vi "runtest initialize fields.vi"(4 "Process SPARTAN SN (F)":bool, 6 "User/Station":T8, 7 "POST (empty)":T6, 8 "error in (no error)":errorcluster, 9 "ProcessNextItem? (f)":bool, 10 "Test Sequence ID":string, 11 "Connection Refnum":T7) -> (0 "error out":errorcluster, 1 "Fields / Results":T5, 2 "dup Test Sequence ID":string, 3 "Connection Refnum":T7, 5 "POST out":T6)   [LabVIEW 2011]
uses:
  Addons/internet/utils/keyedarr.llb/Keyed Array.ctl
  SI.LIB/ODBC/SQL Controls/Connection Refnum.ctl
  runtest User - Station.ctl
  server/database/Stations/Instruments/Instrument Record.ctl
  server/database/Stations/Step Associations/Step Association Record.ctl
  server/database/Fields/Field Record.ctl
  server/database/Fields/Field DataTypes.ctl
  server/database/Fields/Field NextItem.ctl
  tests/Test Output.ctl
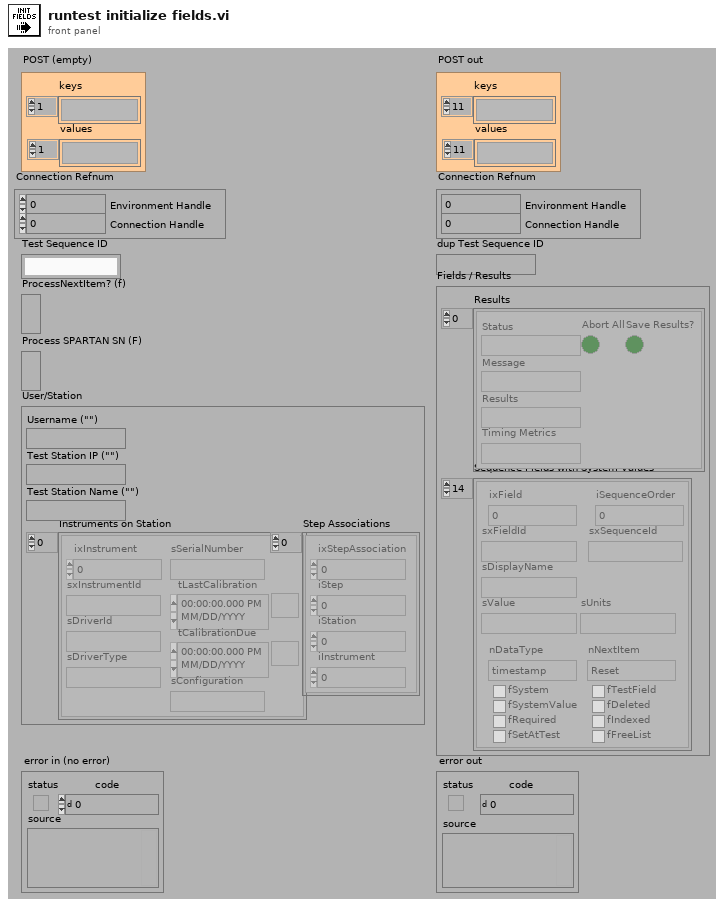
[diagram p1: front panel]
types:
  T1 = typedef "Field Record.ctl" = cluster{"ixField":i32, "iSequenceOrder":i32, "sxFieldId":string, "sxSequenceId":string, "sDisplayName":string, "sValue":string, "sUnits":string, "nDataType":T2, "nNextItem":T3, "fSystem":bool, "fSystemValue":bool, "fRequired":bool, "fSetAtTest":bool, "fTestField":bool, "fDeleted":bool, "fIndexed":bool, "fFreeList":bool}
  T2 = typedef "Field DataTypes.ctl" = enum32{"text", "numeric", "list", "timestamp", "boolean"}
  T3 = typedef "Field NextItem.ctl" = enum32{"Reset", "Retain", "Auto-Increment"}
  T4 = typedef "Test Output.ctl" = cluster{"Status":string, "Message":string, "Results":string, "Abort All":bool, "Save Results?":bool, "Timing Metrics":string}
  T5 = cluster{"Sequence Fields with System Values":T1[], "Results":T4[]}
  T6 = typedef "Keyed Array.ctl" = cluster{"keys":string[], "values":string[]}
  T7 = typedef "Connection Refnum.ctl" = cluster{"Environment Handle":i32, "Connection Handle":i32}
  T8 = typedef "runtest User - Station.ctl" = cluster{"Username (\"\")":string, "Test Station IP (\"\")":string, "Test Station Name (\"\")":string, "Instruments on Station":T9[], "Step Associations":T10[]}
  T9 = typedef "Instrument Record.ctl" = cluster{"ixInstrument":i32, "sxInstrumentId":string, "sDriverId":string, "sDriverType":string, "sSerialNumber":string, "tLastCalibration":timestamp, "tCalibrationDue":timestamp, "sConfiguration":string}
  T10 = typedef "Step Association Record.ctl" = cluster{"ixStepAssociation":i32, "iStep":i32, "iStation":i32, "iInstrument":i32}
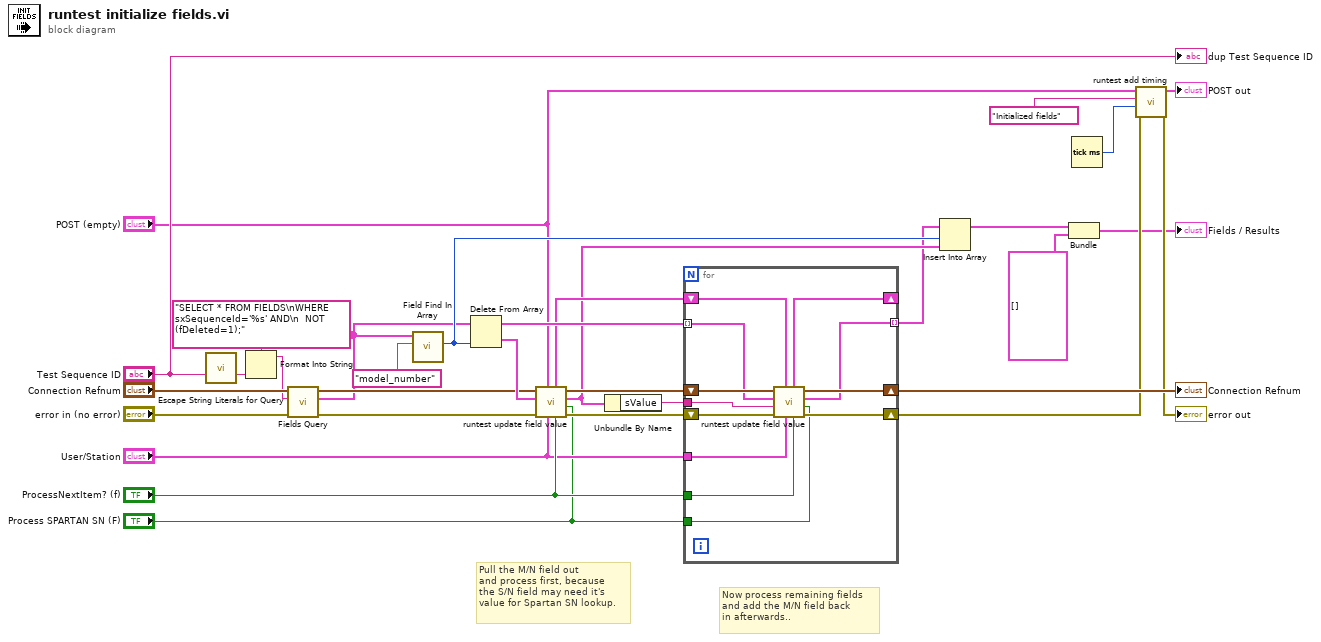
[diagram p0: block diagram]
diagram:
  # "Now process remaining fields\nand add the M/N field back\nin afterwards.."
  # "Pull the M/N field out\nand process first, because\nthe S/N field may need it's\nvalue for Spartan SN lookup."
  n1 = call "Escape String Literals for Query.vi"("String"="Test Sequence ID") -> ("escaped String"=w3:string)  [unwired: 1 in, 13 out]
  n2 = Format Into String(format string="SELECT * FROM FIELDS\nWHERE sxSequenceId='%s' AND\n  NOT (fDeleted=1);" ("User Query"), w3) -> (resulting string=w5:string)  [unwired: 2 in, 1 out]
  n3 = call "Fields Query.vi"("error in (no error)"="error in (no error)", "Query"=w5, "Connection Refnum"="Connection Refnum") -> ("error out"=w1:errorcluster, "Fields"=w7:T1[], "Connection Refnum"=w8:T7)  [unwired: 1 in, 5 out]
  n4 = call "Field Find In Array.vi"("FieldID or Display Name(\"\")"="model_number", "Field Array"=w7) -> ("Index"=w31:i32)  [unwired: 1 in, 8 out]
  n5 = Delete From Array(array=w7, index=w31) -> (deleted portion=w23:T1, array with subset deleted=w30:T1[])  [unwired: 1 in]
  n6 = call "runtest update field value.vi"("Process SPARTAN SN (F)"="Process SPARTAN SN (F)", "ProcessNextItem? (f)"="ProcessNextItem? (f)", "User/Station"="User/Station", "POST (empty)"="POST (empty)", "error in (no error)"=w1, "Field"=w23, "Connection Refnum"=w8) -> ("error out"=w29:errorcluster, "updated Field"=w26:T1, "Connection Refnum"=w28:T7, "remaining POST"=w27:T6)  [unwired: 1 in]
  n7 = Unbundle By Name(w26) -> ("sValue"=w25:string)
  n8 = for {
    tunnel: w30 -> [w35] mode=indexing
    shift-right: [w40] -> _
    shift-left: w27 -> [w41]
    shift-right: [w42] -> w16
    shift-left: w29 -> [w43]
    shift-right: [w38] -> w22
    shift-left: w28 -> [w44]
    tunnel: w25 -> [w39]
    tunnel: [w37] -> w24 mode=indexing
    tunnel: "User/Station" -> [w36]
    tunnel: "ProcessNextItem? (f)" -> [w34]
    tunnel: "Process SPARTAN SN (F)" -> [w33]
    n9 = call "runtest update field value.vi"("Process SPARTAN SN (F)"=w33, "ProcessNextItem? (f)"=w34, "User/Station"=w36, "POST (empty)"=w41, "error in (no error)"=w43, "Model Number (\"\")"=w39, "Field"=w35, "Connection Refnum"=w44) -> ("error out"=w42:errorcluster, "updated Field"=w37:T1, "Connection Refnum"=w38:T7, "remaining POST"=w40:T6)
  }
  "Connection Refnum" <- w22
  n10 = Insert Into Array(array=w24, index=w31, new element=w26) -> (w14:T1[])
  n11 = Bundle(w14, "Test Step Outputs"=T4[] []) -> (→"Fields / Results":cluster{T1[], "Test Step Outputs":T4[]})  [unwired: 1 out]
  n12 = Tick Count (ms)() -> (millisecond timer value=w17:u32)
  n13 = call "runtest add timing.vi"("error in (no error)"=w16, "Start Tick, ms (0)"=w17, "Function (\"\")"="Initialized fields", "POST (empty)"="POST (empty)") -> ("error out"=→"error out":errorcluster, "POST out"=→"POST out":T6)  [unwired: 6 out]
  "dup Test Sequence ID" <- "Test Sequence ID"
